vi "recipeScript userParamStrToArray.vi"(2 "error in (no error)":errorcluster, 3 "recipeScript":string) -> (0 "error out":errorcluster, 1 "userParam":string[][](array[string]))   [LabVIEW 2018]
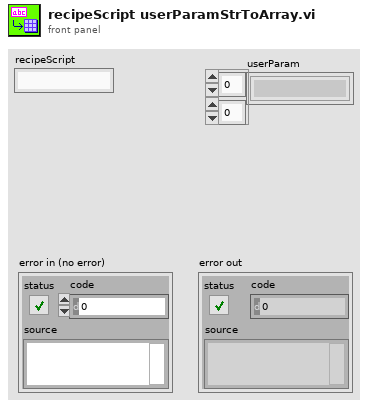
[diagram p1: front panel]
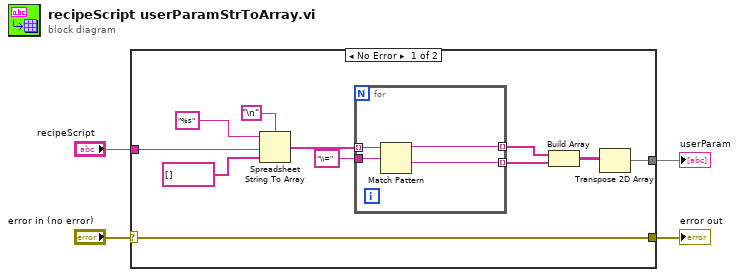
[diagram p0: block diagram]
diagram:
  n1 = case shown="No Error" "error in (no error)" {
    selector: "error in (no error)" -> [w10 w20]
    tunnel: [w11 _] -> w4
    tunnel: [w10 w20] -> w3
    tunnel: "recipeScript" -> [w6 _]
    frame No Error {
      n2 = Spreadsheet String To Array(delimiter (Tab)="\n", format string="%s", spreadsheet string=w6, array type (2D Dbl)=string[] []) -> (array=w5:string[])
      n3 = for {
        tunnel: w5 -> [w19] mode=indexing
        tunnel: "\\=" -> [w18]
        tunnel: [w17] -> w14 mode=indexing
        tunnel: [w16] -> w13 mode=indexing
        n4 = Match Pattern(string=w19, regular expression=w18) -> (before substring=w16:string, after substring=w17:string)  [unwired: 1 in, 2 out]
      }
      n5 = Build Array(w13, w14) -> (w15:string[][])
      n6 = Transpose 2D Array(2D array=w15) -> (transposed array=w11:string[][])
    }
    frame Error {
    }
  }
  "userParam" <- w4
  "error out" <- w3
